vi "write_record.vi"   [LabVIEW 2019]
types:
  T1 = enum16{"open", "replace", "create", "open or create", "replace or create", "replace or create with confirmation"}
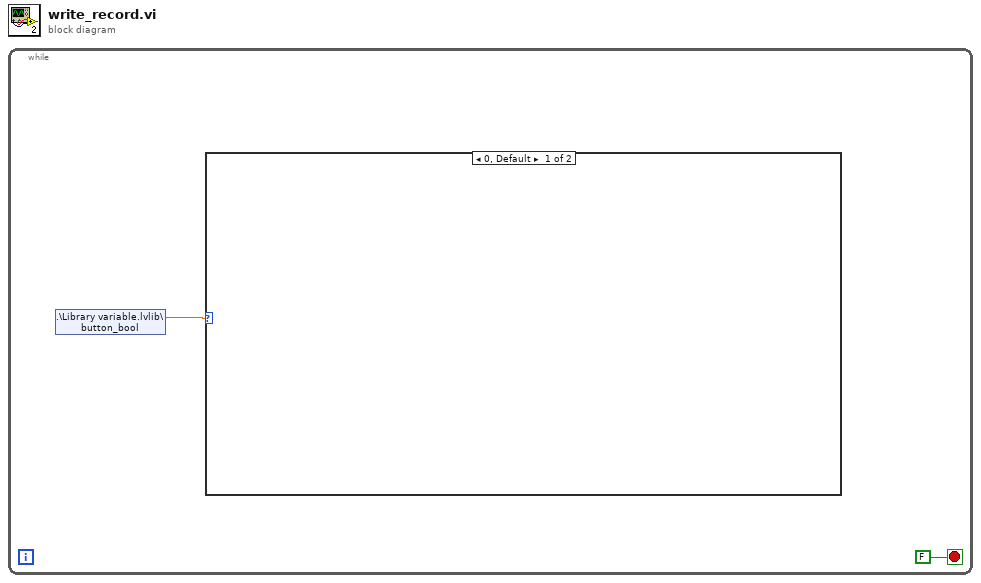
[diagram p0: block diagram]
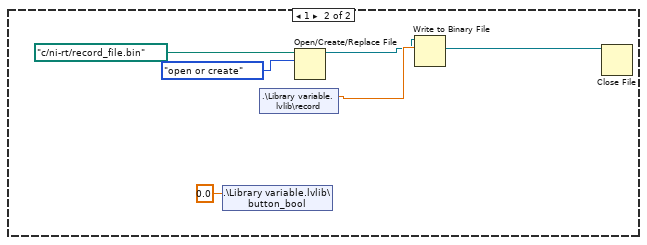
[diagram p2: hidden frame]
diagram:
  n1 = while {
    stop <- FALSE stop-if-true
    n2 = shared-variable ".\\Library variable.lvlib\\button_bool"() -> (w2:dbl)  [unwired: 1 in, 1 out]
    n3 = case shown="0, Default" w2 {
      frame 0, Default {
      }
      frame 1 {
        n4 = shared-variable ".\\Library variable.lvlib\\button_bool"(0.0 ("button_bool")) -> ()  [unwired: 1 in, 1 out]
        n5 = shared-variable ".\\Library variable.lvlib\\record"() -> (w8:dbl)  [unwired: 1 in, 1 out]
        n6 = Open/Create/Replace File(file path (use dialog)=path "c:/ni-rt/record_file.bin", operation (0:open)=T1."open or create") -> (refnum out=w7:refnum<file>)  [unwired: 4 in, 2 out]
        n7 = Write to Binary File(file (use dialog)=w7, data=w8) -> (refnum out=w6:refnum<file>)  [unwired: 4 in, 2 out]
        n8 = Close File(refnum=w6) -> ()  [unwired: 1 in, 2 out]
      }
    }
  }
